vi "decode.vi"() -> ()   [LabVIEW 2010]
panel:
  out "有无后续帧":bool
  out "数据处理状态":bool
  out "数据字符串输出":string
  out "数据类型":string
  in  "字符串输入":string="6801000000000068910600010102"
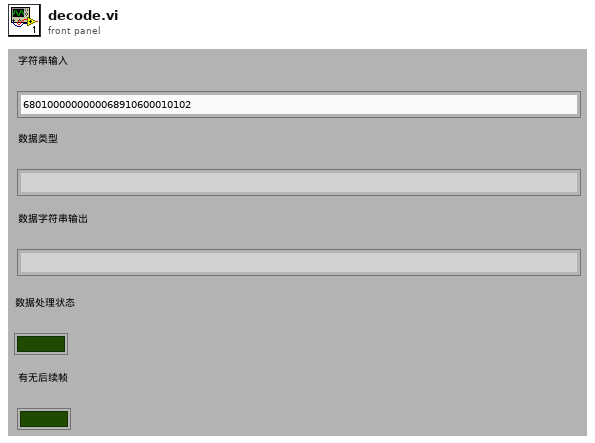
[diagram p1: front panel]
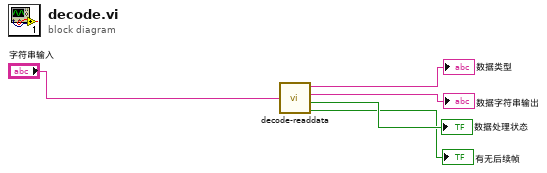
[diagram p0: block diagram]
diagram:
  n1 = call "decode-readdata.vi"("字符串输入"="字符串输入") -> ("有无后续帧"=→"有无后续帧":bool, "数据处理状态"=→"数据处理状态":bool, "数据字符串"=→"数据字符串输出":string, "类型字符串"=→"数据类型":string)
